vi "Map From Bitmask.vi"(8 "error in (no error)":errorcluster, 10 "Bitmask":u64, 11 "ElectrodeGrid in":refnum<class "ElectrodeGrid.lvclass">) -> (0 "error out":errorcluster, 2 "Elec Grid Output":bool[][](array[boolean]), 3 "ElectrodeGrid out":refnum<class "ElectrodeGrid.lvclass">)   [LabVIEW 2017, in "ElectrodeGrid.lvclass"]
doc: "From a 64-bit input, this VI will map the object's boolean electrode grid.\n\nThe bitmask map which describes each grid element's HV channel connection comes from the object's property."
uses:
  ElectrodeGrid.lvclass
  ElectrodeGrid.lvclass/ElectrodeGrid.ctl
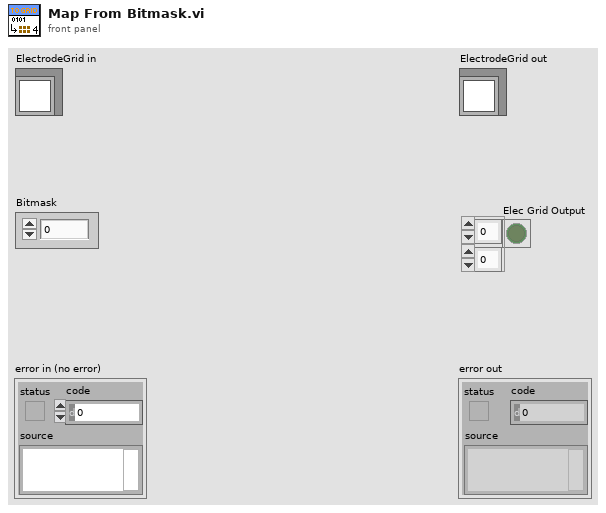
[diagram p1: front panel]
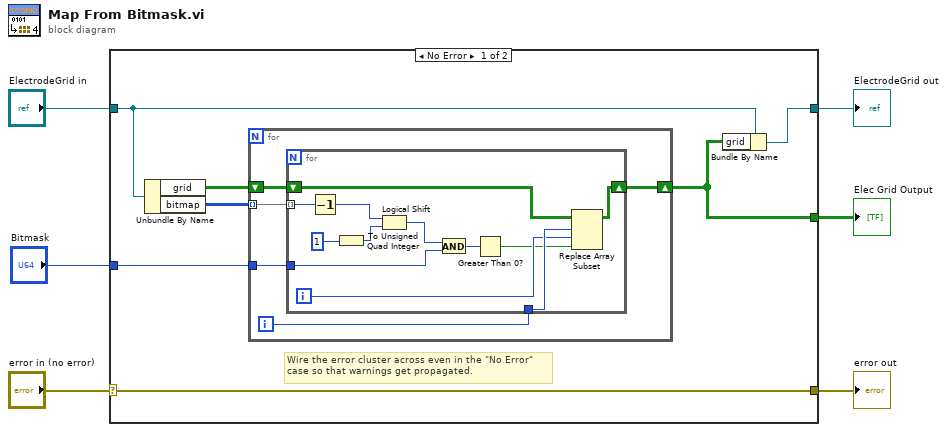
[diagram p0: block diagram]
diagram:
  n1 = case shown="No Error" "error in (no error)" {
    selector: "error in (no error)" -> [w13 w32]
    tunnel: [w13 w32] -> w5
    tunnel: [w11 w31] -> w3
    tunnel: "ElectrodeGrid in" -> [w12 w31]
    tunnel: "Bitmask" -> [w9 _]
    tunnel: [w7 _] -> w1
    frame No Error {
      # "Wire the error cluster across even in the \"No Error\"\ncase so that warnings get propagated."
      n2 = Unbundle By Name(w12) -> ("grid"=w8:bool[][], "bitmap"=w10:u8[][])
      n3 = for {
        tunnel: w10 -> [w18] mode=indexing
        tunnel: w9 -> [w17]
        shift-right: [w15] -> w7
        shift-left: w8 -> [w14]
        i -> [w16]
        n4 = for {
          tunnel: w18 -> [w30] mode=indexing
          tunnel: w17 -> [w28]
          tunnel: w16 -> [w23]
          shift-right: [w20] -> w15
          shift-left: w14 -> [w19]
          i -> [w22]
          n5 = Decrement(x=w30) -> (x-1=w29:u8)
          n6 = To Unsigned Quad Integer(1:u32 1 ("x")) -> (0:w25:u64)
          n7 = Logical Shift(y=w29, x=w25) -> (x << y=w27:u64)
          n8 = And(x=w27, y=w28) -> (x .and. y?=w24:u64)
          n9 = Greater Than 0?(x=w24) -> (x > 0?=w21:bool)
          n10 = Replace Array Subset(array=w19, new element=w21, index (row)=w23, index (col)=w22) -> (w20:bool[][])
        }
      }
      n11 = Bundle By Name(cluster=w12, "grid"=w7) -> (w11:refnum<class "ElectrodeGrid.lvclass">)
    }
    frame Error {
    }
  }
  "error out" <- w5
  "ElectrodeGrid out" <- w3
  "Elec Grid Output" <- w1
